vi "LevelString.vi"(8 "error in (no error)":errorcluster, 11 "Level":T1=enum."INFO") -> (0 "error out":errorcluster, 3 "LevelName":string)   [LabVIEW 2026, in "Lumberjack.lvlib"]
uses:
  Lumberjack.lvlib
  Types/Severity.ctl
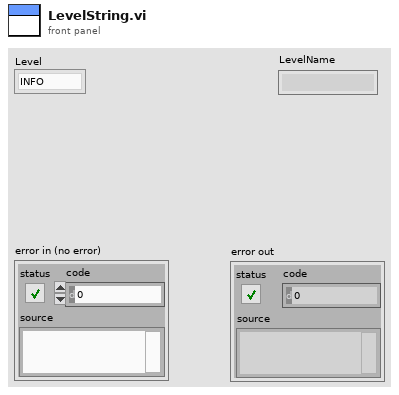
[diagram p1: front panel]
types:
  T1 = typedef "Lumberjack.lvlib/Severity.ctl" = enum16{"OFF", "FATAL", "ERROR", "WARN", "INFO", "DEBUG", "TRACE", "ALL"}
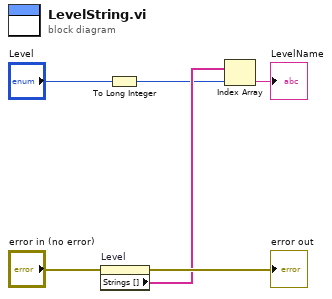
[diagram p0: block diagram]
diagram:
  n1 = property on="Level" class="Enum (strict)"(error in="error in (no error)") -> (error out=→"error out":errorcluster, "Strings []"=w4:string[])  [unwired: 1 in, 1 out]
  n2 = To Long Integer(number="Level") -> (32bit integer=w1:i32)
  n3 = Index Array(array=w4, index=w1) -> (element=→"LevelName":string)
